vi "Command Dispatch.vi"(8 "error in (no error)":errorcluster, 10 "GUID-cmd-data":T1, 11 "WS Server in":refnum<class "WS Server.lvclass">) -> (0 "error out":errorcluster, 3 "WS Server out":refnum<class "WS Server.lvclass">)   [LabVIEW 2016, in "WebSocket Networking.lvlib" / "WS Server.lvclass"]
uses:
  <userlib>/Common Components/WebSocket Networking/WS Server/WS Server.lvclass
  <userlib>/Common Components/Common/GUID-command-data.ctl
  <userlib>/Common Components/WebSocket Networking/WS Server/WS Server.lvclass/WS Server.ctl
  <userlib>/Common Components/Controller Messages/Command Dispatch Msg/Command Dispatch Msg.lvclass/Command Dispatch Msg.ctl
  <vilib>/ActorFramework/Message Enqueuer/Message Enqueuer.lvclass/Message Enqueuer.ctl
  <vilib>/ActorFramework/Message Enqueuer/Enqueue.vi
  <userlib>/Common Components/Controller Messages/Command Dispatch Msg/Command Dispatch Msg.lvclass
  C:/Program Files (x86)/National Instruments/LabVIEW 2016/vi.lib/ActorFramework/Message/Message.lvclass
  <vilib>/ActorFramework/Message Priority Queue/Priority Enqueue.vi
  <userlib>/Common Components/Common/Common.lvlib
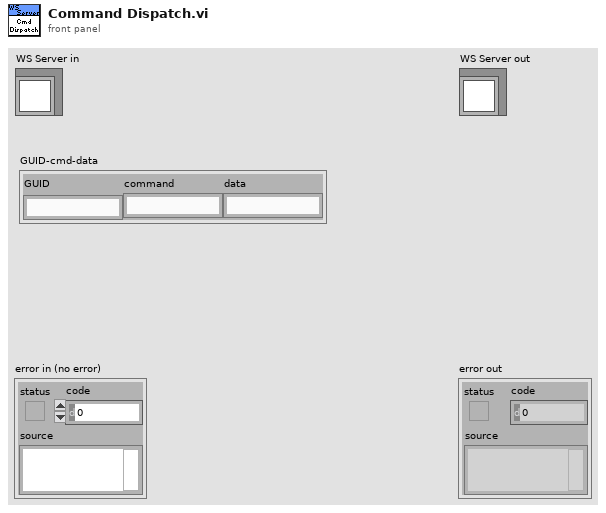
[diagram p1: front panel]
types:
  T1 = typedef "Common.lvlib/GUID-command-data.ctl" = cluster{"GUID":string, "command":string, "data":string}
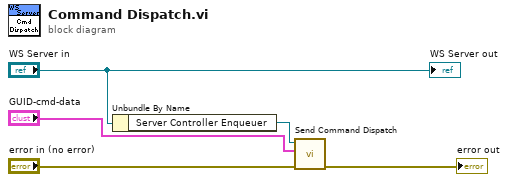
[diagram p0: block diagram]
diagram:
  n1 = Unbundle By Name("WS Server in") -> ("Server Controller Enqueuer"=w2:refnum<class "Message Enqueuer.lvclass">)
  n2 = call <userlib>:"Send Command Dispatch.vi"("error in (no error)"="error in (no error)", "GUID-cmd-data"="GUID-cmd-data", "Message Enqueuer"=w2) -> ("error out"=→"error out":errorcluster)  [unwired: 7 in, 1 out]
  "WS Server out" <- "WS Server in"
